vi "Check_Create.vi"(8 "error in":errorcluster, 11 "PathIn":string) -> (0 "error out":errorcluster, 2 "dup path":path, 3 "PathOut":string)   [LabVIEW 2014, in "Files_OP.lvlib"]
uses:
  Files_OP.lvlib
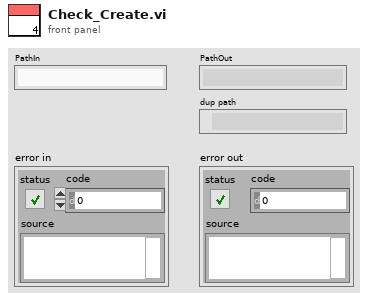
[diagram p1: front panel]
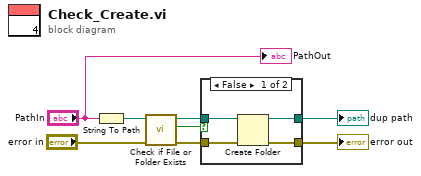
[diagram p0: block diagram]
diagram:
  n1 = String To Path(string="PathIn") -> (path=w4:path)
  n2 = call <vilib>:"Check if File or Folder Exists.vi"("error in (no error)"="error in", "path"=w4) -> ("error out"=w6:errorcluster, "file or folder exists?"=w7:bool, "dup path"=w5:path)  [unwired: 7 in]
  n3 = case shown="False" w7 {
    tunnel: w5 -> [w12 w13]
    tunnel: w6 -> [w11 w14]
    tunnel: [w10 w14] -> w8
    tunnel: [w9 w13] -> w2
    frame False {
      n4 = Create Folder(path (use dialog)=w12, error in=w11) -> (created path=w9:path, error out=w10:errorcluster)  [unwired: 1 in, 1 out]
    }
    frame True {
    }
  }
  "error out" <- w8
  "dup path" <- w2
  "PathOut" <- "PathIn"
